vi "long term plate tap.vi"() -> ()   [LabVIEW 2014]
panel:
  in  "Number of Experiments":i32
  in  "Wait between experiments (s)":dbl
  in  "Hold Time (frames)":i32
  in  "period  (frames)":i32
  in  "Trials Per Voltage":i32
  in  "Array":dbl[](array[numeric])
  in  "Min Voltage":dbl
  out "Frames":i32
  in  "Transfer and Run Date Folder After Experiment":bool
  in  "SSH user name":string
  in  "SSH password":string
  in  "Wait before recording (s)":dbl
  in  "Tags":string
  in  "Start Recording":bool
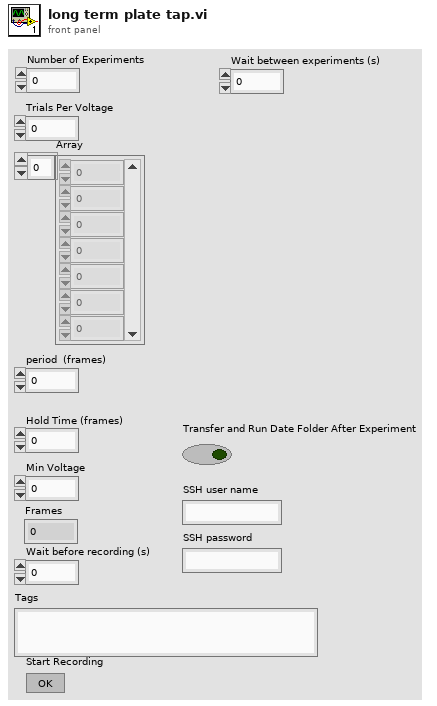
[diagram p1: front panel]
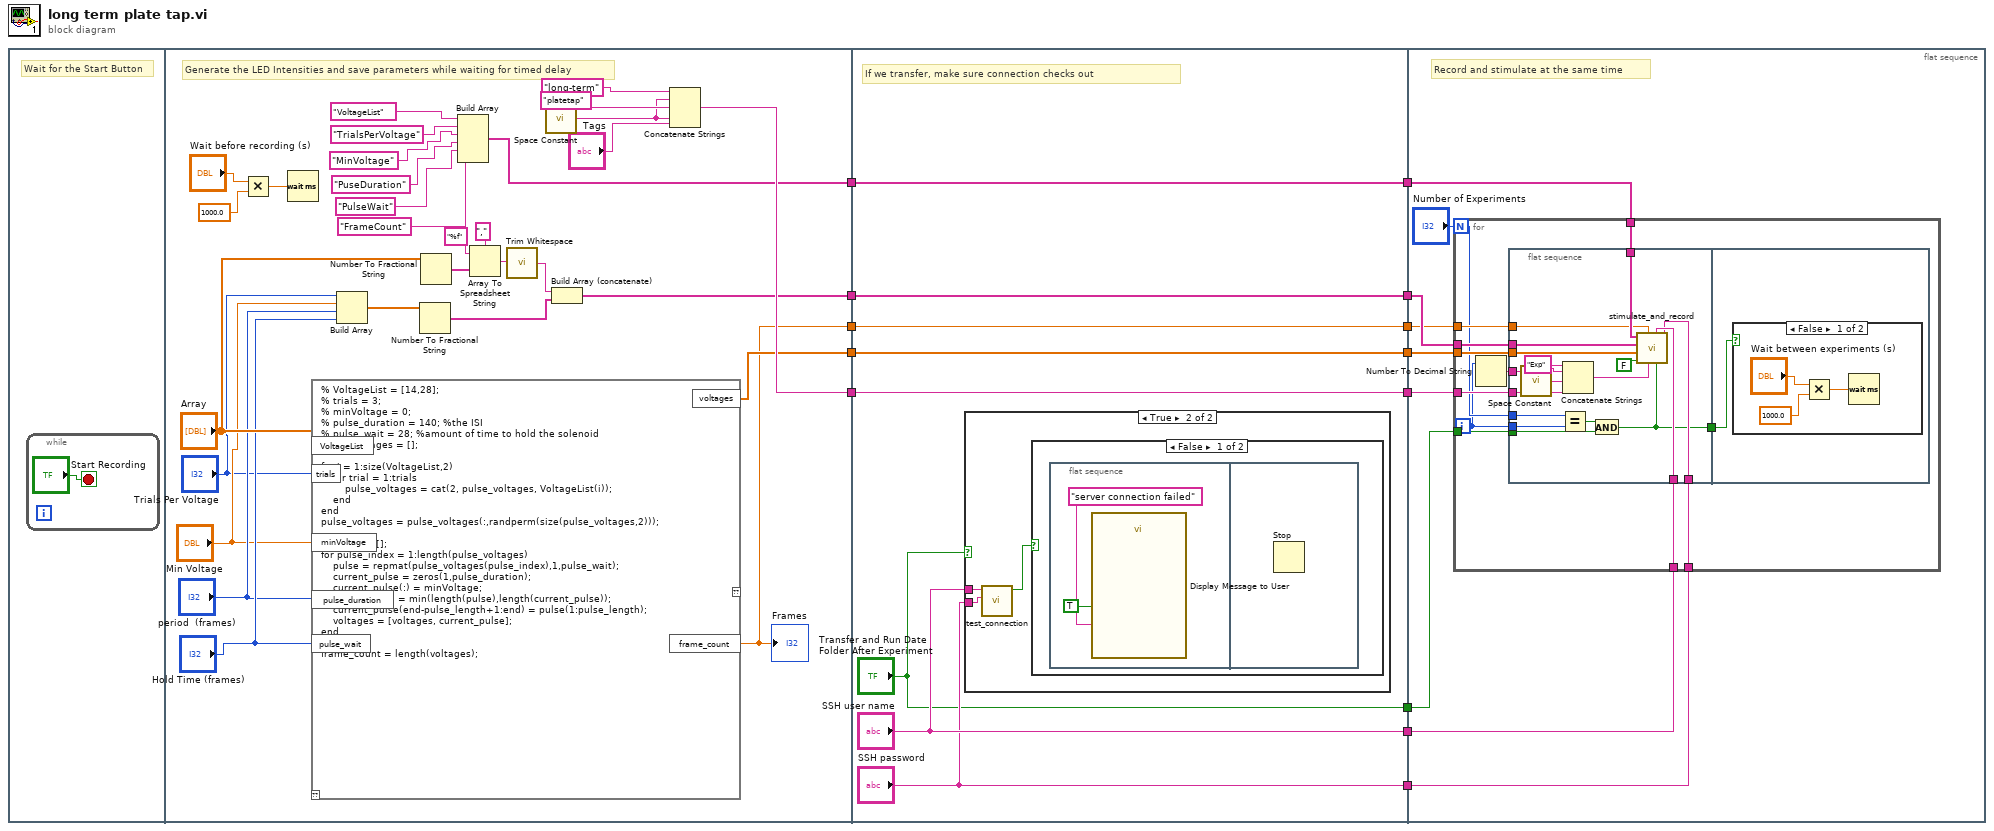
[diagram p0: block diagram]
diagram:
  n1 = flat-sequence {
    tunnel: [w42] -> w13
    tunnel: [w26] -> w11
    tunnel: [w36] -> w9
    tunnel: [w18] -> w7
    tunnel: [w17] -> w5
    tunnel: w13 -> [w52]
    tunnel: [w52] -> w12
    tunnel: w11 -> [w51]
    tunnel: [w51] -> w10
    tunnel: w9 -> [w50]
    tunnel: [w50] -> w8
    tunnel: w7 -> [w49]
    tunnel: [w49] -> w6
    tunnel: w5 -> [w48]
    tunnel: [w48] -> w4
    tunnel: ["SSH user name"] -> w3
    tunnel: ["SSH password"] -> w2
    tunnel: ["Transfer and Run Date Folder After Experiment"] -> w1
    tunnel: w12 -> [w66]
    tunnel: w10 -> [w65]
    tunnel: w8 -> [w64]
    tunnel: w6 -> [w63]
    tunnel: w4 -> [w62]
    tunnel: w3 -> [w61]
    tunnel: w2 -> [w60]
    tunnel: w1 -> [w59]
    frame #0 {
      # "Wait for the Start Button"
      n2 = while {
        stop <- "Start Recording" stop-if-true
      }
    }
    frame #1 {
      # "Generate the LED Intensities and save parameters while waiting for timed delay"
      n3 = Multiply(x="Wait before recording (s)", y=1000.0) -> (x*y=w40:dbl)
      n4 = Wait (ms)(milliseconds to wait=w40) -> ()  [unwired: 1 out]
      n5 = script code="% VoltageList = [14,28];\n% trials = 3;\n% minVoltage = 0;\n% pulse_duration = 140; %the ISI\n% pulse_wait = 28; %amount of time to hold the solenoid\npulse_voltages = [];\n\nfor i = 1:size(VoltageList,2)\n    for trial = 1:trials\n        pulse_voltages = cat(2, pulse_voltages, VoltageList(i));\n    end\nend\npulse_voltages = pulse_voltages(:,randperm(size(pulse_voltages,2)));\n\nvoltages = [];\nfor pulse_index = 1:length(pulse_voltages)\n    pulse = repmat(pulse_voltages(pulse_index),1,pulse_wait);\n    current_pulse = zeros(1,pulse_duration);\n    current_pulse(:) = minVoltage;\n    pulse_length = min(length(pulse),length(current_pulse));\n    current_pulse(end-pulse_length+1:end) = pulse(1:pulse_length);\n    voltages = [voltages, current_pulse];\nend\n\nframe_count = length(voltages);"("pulse_duration"="period  (frames)", "trials"="Trials Per Voltage", "minVoltage"="Min Voltage", "VoltageList"="Array", "pulse_wait"="Hold Time (frames)") -> ("voltages"=w18:dbl[], "frame_count"=w17:dbl)  [unwired: 1 in, 1 out]
      "Frames" <- w17
      n6 = Build Array("Trials Per Voltage", "Min Voltage", "period  (frames)", "Hold Time (frames)") -> (w25:dbl[])
      n7 = Number To Fractional String(number=w25) -> (F-format string=w37:string[])  [unwired: 3 in]
      n8 = Number To Fractional String(number="Array") -> (F-format string=w24:string[])  [unwired: 3 in]
      n9 = Build Array("VoltageList", "TrialsPerVoltage", "MinVoltage", "PuseDuration", "PulseWait", "FrameCount") -> (w26:string[])
      n10 = Array To Spreadsheet String(delimiter (Tab)=",", array=w24, 3:"%f") -> (spreadsheet string=w34:string)
      n11 = call <vilib>:"Trim Whitespace.vi"("string"=w34) -> ("trimmed string"=w33:string)  [unwired: 1 in]
      n12 = call <vilib>:"Space Constant.vi"() -> ("String"=w16:string)
      n13 = Build Array (concatenate)(w33, w37) -> (w36:string[])
      n14 = Concatenate Strings("long-term", w16, "platetap", w16, "Tags") -> (w42:string)
    }
    frame #2 {
      # "If we transfer, make sure connection checks out"
      n15 = case shown="True" "Transfer and Run Date Folder After Experiment" {
        tunnel: "SSH user name" -> [_ w54]
        tunnel: "SSH password" -> [_ w53]
        frame False {
        }
        frame True {
          n16 = call "test_connection.vi"("Username"=w54, "Password"=w53) -> ("Connection Successful"=w55:bool)  [unwired: 7 in]
          n17 = case shown="False" w55 {
            frame False {
              n18 = flat-sequence {
                frame #0 {
                  n19 = call "Display Message to User"("Enable"=TRUE, "Message"="server connection failed") -> ()  [unwired: 8 in, 2 out]
                }
                frame #1 {
                  n20 = Stop() -> ()  [unwired: 1 in]
                }
              }
            }
            frame True {
            }
          }
        }
      }
    }
    frame #3 {
      # "Record and stimulate at the same time"
      n21 = for {
        N: "Number of Experiments" -> [w69]
        tunnel: w66 -> [w78]
        tunnel: w65 -> [w77]
        tunnel: w64 -> [w76]
        tunnel: w63 -> [w75]
        tunnel: w62 -> [w74]
        tunnel: w61 -> [w73]
        tunnel: w60 -> [w72]
        tunnel: w59 -> [w71]
        i -> [w67]
        n22 = Number To Decimal String(number=w67) -> (decimal integer string=w68:string)  [unwired: 1 in]
        n23 = flat-sequence {
          tunnel: w78 -> [w83]
          tunnel: w77 -> [w94]
          tunnel: w76 -> [w93]
          tunnel: w75 -> [w92]
          tunnel: w74 -> [w91]
          tunnel: w73 -> [w90]
          tunnel: w72 -> [w89]
          tunnel: w71 -> [w88]
          tunnel: w69 -> [w86]
          tunnel: w67 -> [w85]
          tunnel: [w84] -> w70
          tunnel: w68 -> [w80]
          tunnel: w70 -> [w96]
          frame #0 {
            n24 = call <vilib>:"Space Constant.vi"() -> ("String"=w81:string)
            n25 = Equal?(x=w86, y=w85) -> (x = y?=w87:bool)
            n26 = Concatenate Strings("Exp", w80, w81, w83) -> (w82:string)
            n27 = And(x=w87, y=w88) -> (x .and. y?=w84:bool)
            n28 = call "stimulate_and_record.vi"("SSH password"=w89, "Transfer and Run Date Folder After Experiment"=w84, "SSH user name"=w90, "Tags"=w82, "Frames"=w91, "Convert Power to Voltage"=FALSE, "voltages/power"=w92, "parameters"=w93, "parameters headers"=w94) -> ()  [unwired: 3 in]
          }
          frame #1 {
            n29 = case shown="False" w96 {
              frame False {
                n30 = Multiply(x="Wait between experiments (s)", y=1000.0) -> (x*y=w98:dbl)
                n31 = Wait (ms)(milliseconds to wait=w98) -> ()  [unwired: 1 out]
              }
              frame True {
              }
            }
          }
        }
      }
    }
  }
